vi "GEA2 Message Received Event Handler.vi"(4 "Recv Data":refnum<user-event>, 5 "Event Data":T1, 6 "Control Ref":refnum<k24>, 7 "Event Common Data":T2) -> ()   [LabVIEW 2023, in "GEA2_Toolkit.lvlib"]
doc: "This subVI is executed upon receiving an event (GEA2 data). It parses the data and returns: source, destination, command, length, CRC, and data. The inputs CANNOT be modified."
uses:
  library/GEA2_Toolkit.lvlib
  D:/Common/LabVIEW GEA2 Toolkit/source/GEA3 DLL Source/GeaCommunication.dll
  source/GEA3 DLL Source/GeaCommunication.dll
  type defs/Data Out.ctl
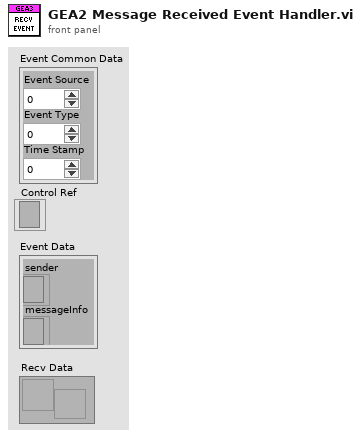
[diagram p1: front panel]
types:
  T1 = cluster{"sender":refnum<k24>, "messageInfo":refnum<k24>}
  T2 = cluster{"Event Source":i32, "Event Type":u32, "Time Stamp":u32}
  T3 = typedef "GEA2_Toolkit.lvlib/Data Out.ctl" = cluster{"Source":u8, "Destination":u8, "Command":u8, "Length":u8, "CRC":u16, "Message":string}
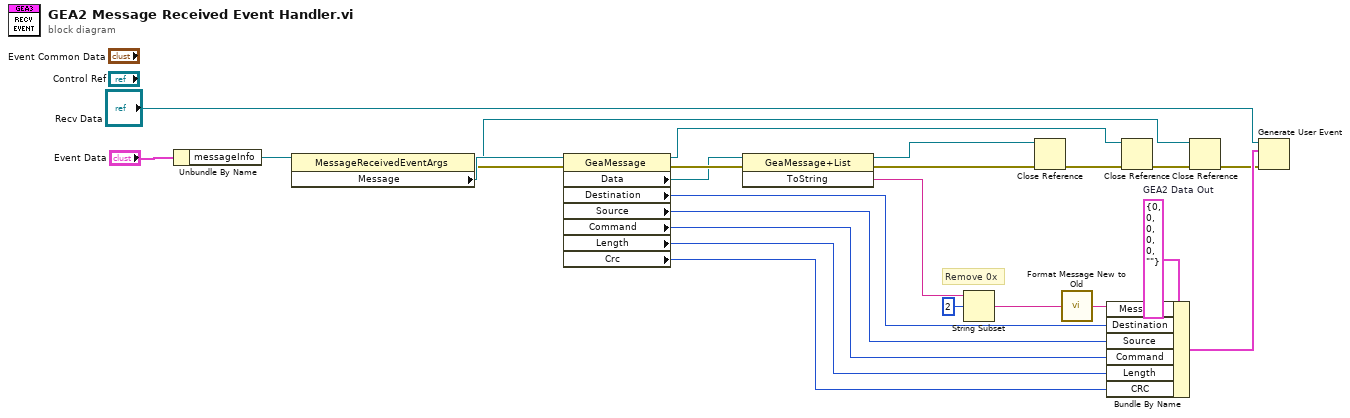
[diagram p0: block diagram]
diagram:
  w24 = T3 {"Source"=0, "Destination"=0, "Command"=0, "Length"=0, "CRC"=0, "Message"=""}  # GEA2 Data Out
  # "Remove 0x"
  n1 = Unbundle By Name("Event Data") -> ("messageInfo"=w22:refnum<k24>)
  n2 = property class="MessageReceivedEventArgs"(reference=w22) -> (reference out=w5:refnum<k24>, error out=w13:errorcluster, "Message"=w19:refnum<k24>)  [unwired: 1 in]
  n3 = property class="GeaMessage"(reference=w19, error in=w13) -> (reference out=w6:refnum<k24>, error out=w9:errorcluster, "Data"=w4:refnum<k24>, "Destination"=w18:u8, "Source"=w17:u8, "Command"=w16:u8, "Length"=w15:u8, "Crc"=w14:u16)
  n4 = invoke class="GeaMessage+List" method="ToString"(reference=w4, error in=w9) -> (reference out=w7:refnum<k24>, error out=w8:errorcluster, "ToString"=w3:string)  [unwired: 1 in]
  n5 = String Subset(string=w3, offset (0)=2) -> (substring=w1:string)  [unwired: 1 in]
  n6 = Close Reference(reference=w7, error in (no error)=w8) -> (error out=w21:errorcluster)
  n7 = call "Format Message New to Old.vi"("Raw Message In"=w1) -> ("Conv Message Out"=w10:string)  [unwired: 14 in]
  n8 = Bundle By Name(cluster=w24, "Message"=w10, "Destination"=w18, "Source"=w17, "Command"=w16, "Length"=w15, "CRC"=w14) -> (w23:T3)
  n9 = Close Reference(reference=w6, error in (no error)=w21) -> (error out=w12:errorcluster)
  n10 = Close Reference(reference=w5, error in (no error)=w12) -> (error out=w11:errorcluster)
  n11 = Generate User Event(user event="Recv Data", event data cluster=w23, error in=w11) -> ()  [unwired: 1 in, 2 out]
